vi "FirstRunTest.vi"(11 "Array":string[](array[string])) -> (2 "Message to log to console":string, 3 "exit code":i32)   [LabVIEW 2018]
uses:
  <vilib>/Utility/error.llb/DialogType.ctl
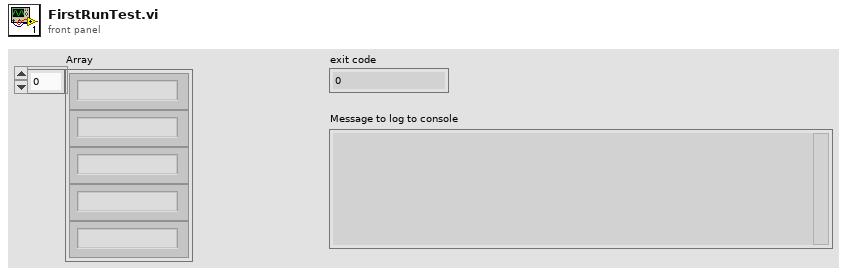
[diagram p1: front panel]
types:
  T1 = typedef "DialogType.ctl" = u16
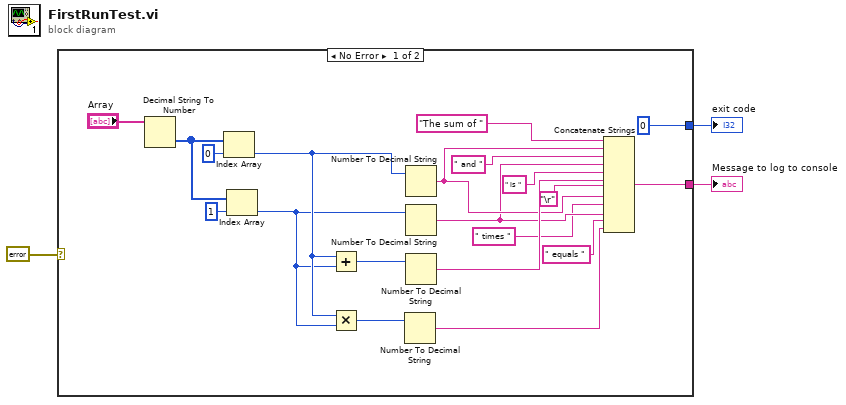
[diagram p0: block diagram]
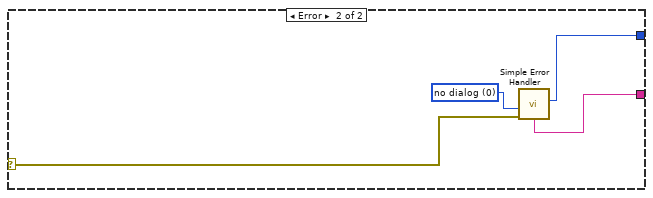
[diagram p2: hidden frame]
diagram:
  n1 = case shown="No Error" errorcluster {"status"=FALSE, "code"=0, "source"=""} ("error IO") {
    selector: errorcluster {"status"=FALSE, "code"=0, "source"=""} ("error IO") -> [_ w27]
    tunnel: [0 ("exit code") w25] -> w3
    tunnel: [w13 w24] -> w2
    frame No Error {
      n2 = Decimal String To Number(string="Array") -> (number=w20:i32[])  [unwired: 2 in, 1 out]
      n3 = Index Array(array=w20, index=0) -> (element=w12:i32)
      n4 = Index Array(array=w20, index=1) -> (element=w11:i32)
      n5 = Add(x=w12, y=w11) -> (x+y=w21:i32)
      n6 = Multiply(x=w12, y=w11) -> (x*y=w10:i32)
      n7 = Number To Decimal String(number=w10) -> (decimal integer string=w4:string)  [unwired: 1 in]
      n8 = Number To Decimal String(number=w12) -> (decimal integer string=w8:string)  [unwired: 1 in]
      n9 = Number To Decimal String(number=w11) -> (decimal integer string=w7:string)  [unwired: 1 in]
      n10 = Number To Decimal String(number=w21) -> (decimal integer string=w22:string)  [unwired: 1 in]
      n11 = Concatenate Strings("The sum of " ("string"), w8, " and " ("string"), w7, " is " ("string"), w22, "\r", w8, " times " ("string"), w7, " equals " ("string"), w4) -> (w13:string)
    }
    frame Error {
      w26 = T1 0 items=["no dialog", "OK message", "continue or stop message", "OK message + warnings", "continue/stop + warnings"] ("type of dialog (OK msg:1)")
      n12 = call <vilib>:"Simple Error Handler.vi"("type of dialog (OK msg:1)"=w26, "error in (no error)"=w27) -> ("code out"=w25:i32, "message"=w24:string)  [unwired: 3 in, 3 out]
    }
  }
  "exit code" <- w3
  "Message to log to console" <- w2
